vi "usrp_tx.vi"() -> ()   [LabVIEW 2014]
uses:
  <vilib>/addons/Modulation/Analog/support/mod_Set Error Source.vi
  var_stop.vi
  <vilib>/addons/Modulation/Digital/Support/Common/Validators/mod_Generate Filter Coefficients Validate.vi
  <vilib>/addons/Modulation/Digital/General/subVIs/mod_Generate Filter Coefficients.vi
  <vilib>/addons/Modulation/Digital/General/MT Apply Pulse Shaping Filter (Generic).vi
  <instrlib>/niUSRP/niUSRP Write Tx Data (CDB Cluster).vi
  <vilib>/addons/Modulation/niDMT.lvlib
panel:
  out "error out":errorcluster
  in  "DPSK type":enum16{"binary", "quadrature"}(ring)=enum."quadrature"
  in  "Send Text":bool
  in  "Text to send":string="This is a point-to-point link prototype with synchronization algorithm implemented and is developed by Teng-Hui Huang, Netwrok  Information and Communications Laboratory, NTU Taiwan.\n\nQuick start:\n1. Connect your PC to a USRP.\n2. Run usrp_tx.vi.\n3. Run usrp_rx.vi.\n4. Press \"Send Text\"\n\nFor any issues please send me an e-mail:\nhui811116@outlook.com\n\nTeng-Hui Huang\n2017.11.19"
  in  "System Stop":bool
  in  "Enabled Channels":string(combo)="0"
  in  "Timebase Clock Source":string(combo)="Internal"
  in  "Frequency Source":string(combo)="Internal"
  out "coerced gain":dbl format="%#_6f"
  out "coerced carrier frequency":dbl=100000.0 format="%#_6p"
  out "coerced IQ rate":dbl=100000.0 format="%#_6p"
  in  "active antenna":string="TX1"
  in  "gain":dbl=10.0 format="%#_6f"
  in  "carrier frequency":dbl=915000000.0 format="%#_6p"
  in  "device names":refnum<k15>="192.168.10.3"
  in  "IQ rate":dbl=1000000.0 format="%#_6p"
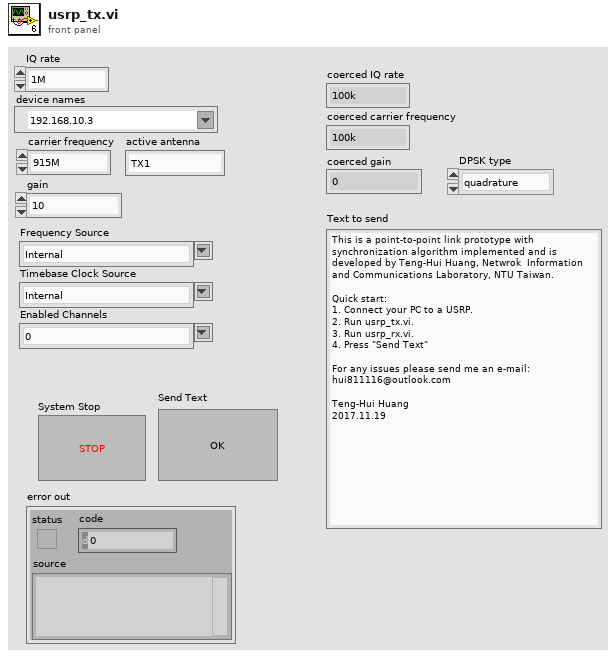
[diagram p1: front panel]
types:
  T1 = enum16{"none", "Raised Cosine", "Root Raised Cos", "Gaussian"}
  T2 = enum16{"FSK", "PSK", "QAM", "MSK", "PAM", "ASK", "CPM"}
  T3 = typedef "niAMT.lvlib/Complex Data Waveform.ctl" = cluster{"t0":dbl, "dt":dbl, "Y":cdb[]}
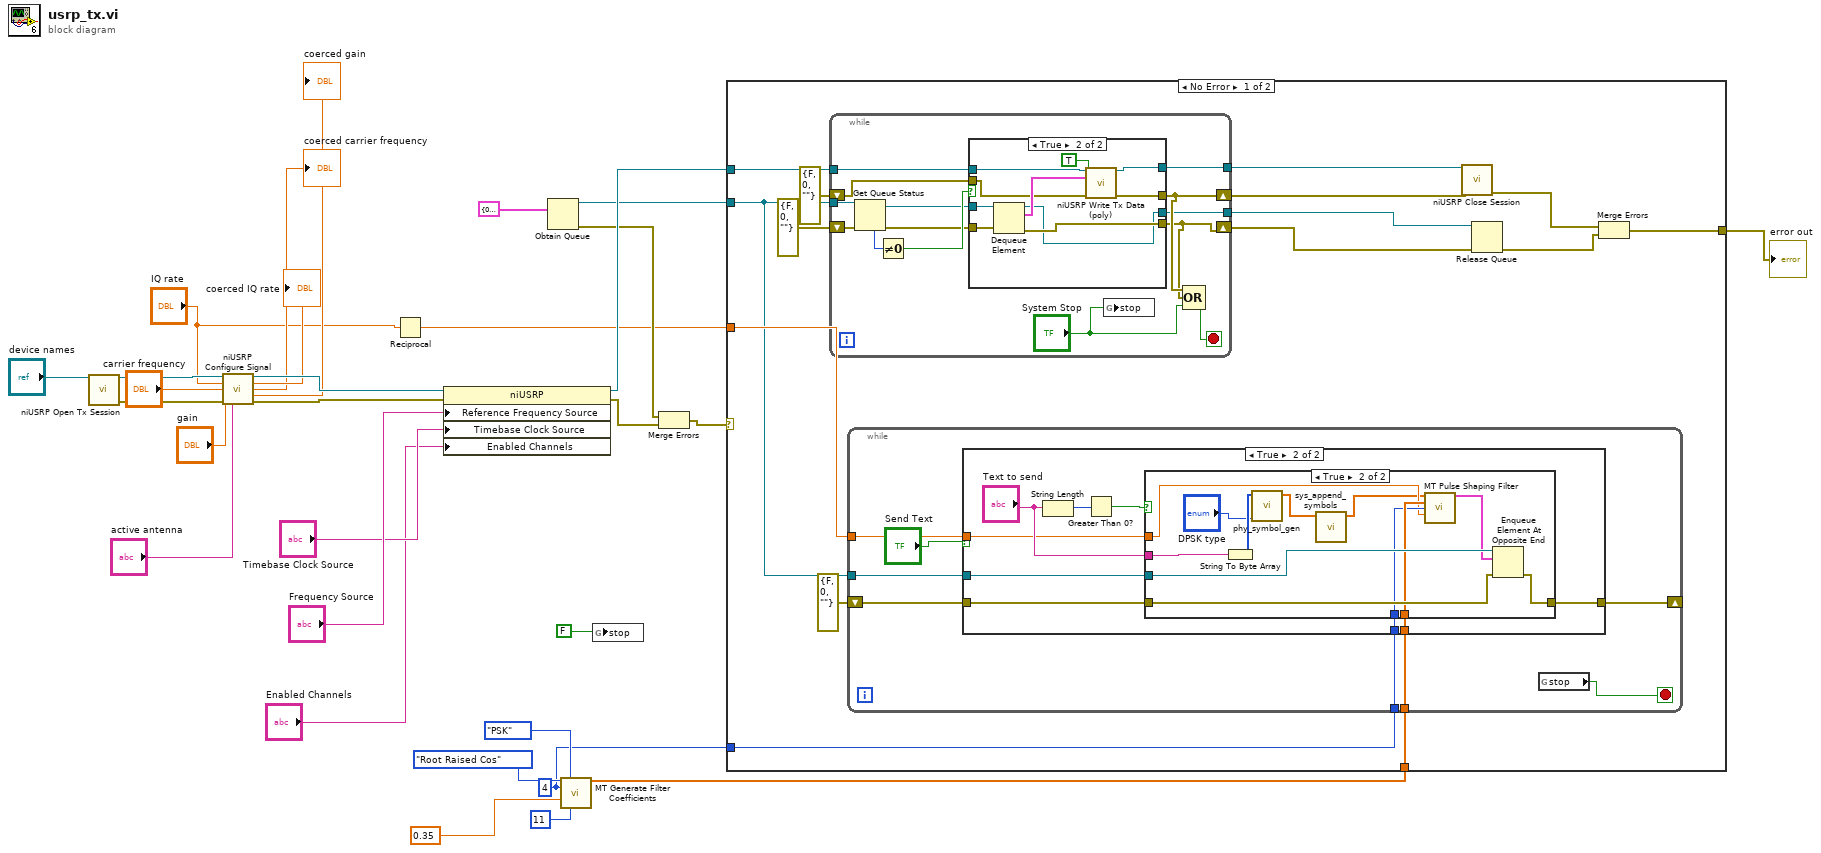
[diagram p0: block diagram]
diagram:
  w2 = 4 ("pulse shaping samples per symbol (16)")
  n1 = call <instrlib>:"niUSRP Open Tx Session.vi"("device names"="device names") -> ("session handle out"=w30:refnum<k15>, "error out"=w29:errorcluster)  [unwired: 13 in]
  n2 = call <instrlib>:"niUSRP Configure Signal.vi"("session handle"=w30, "IQ rate"="IQ rate", "carrier frequency"="carrier frequency", "gain"="gain", "error in (no error)"=w29, "active antenna"="active antenna") -> ("session handle out"=w24:refnum<k15>, "coerced IQ rate"=→"coerced IQ rate":dbl, "coerced carrier frequency"=→"coerced carrier frequency":dbl, "coerced gain"=→"coerced gain":dbl, "error out"=w23:errorcluster)  [unwired: 5 in]
  n3 = Reciprocal(x="IQ rate") -> (1/x=w9:dbl)
  n4 = property class="niUSRP"(reference=w24, error in=w23, "Reference Frequency Source"="Frequency Source", "Timebase Clock Source"="Timebase Clock Source", "Enabled Channels"="Enabled Channels") -> (reference out=w16:refnum<k15>, error out=w14:errorcluster)
  n5 = Obtain Queue(element data type=cluster{"t0":dbl, "dt":dbl, "Y":cdb[]} {"t0"=0.0, "dt"=1.0, "Y"=[]} ("data")) -> (queue out=w15:refnum<queue>, error out=w13:errorcluster)  [unwired: 4 in, 1 out]
  n6 = call <vilib>:"MT Generate Filter Coefficients.vi"("pulse shaping filter (none)"=T1."Root Raised Cos", "modulation type"=T2."PSK", "pulse shaping samples per symbol (16)"=w2, "filter parameter"=0.35, "filter length (symbols)"=11) -> ("pulse shaping filter coefficients"=w3:dbl[])  [unwired: 8 in, 2 out]
  n7 = global write "var_stop.vi" "stop"(FALSE) -> ()
  n8 = Merge Errors(w13, w14) -> (w12:errorcluster)
  n9 = case shown="No Error" w12 {
    selector: w12 -> [_ w105]
    tunnel: w16 -> [w45 _]
    tunnel: w15 -> [w36 _]
    tunnel: w9 -> [w38 _]
    tunnel: w3 -> [w35 _]
    tunnel: w2 -> [w34 _]
    tunnel: [w31 w105] -> w1
    frame No Error {
      n10 = while {
        tunnel: w45 -> [w84]
        tunnel: w36 -> [w89]
        shift-right: [w80] -> w40
        shift-left: errorcluster {"status"=FALSE, "code"=0, "source"=""} ("error out") -> [w88]
        tunnel: [w83] -> w44
        shift-right: [w81] -> w43
        shift-left: errorcluster {"status"=FALSE, "code"=0, "source"=""} ("error out") -> [w82]
        tunnel: [w78] -> w39
        stop <- w79 stop-if-true
        n11 = Get Queue Status(queue=w89, error in (no error)=w88) -> (queue out=w86:refnum<queue>, error out=w85:errorcluster, # elements in queue=w90:i32)  [unwired: 1 in, 5 out]
        n12 = Not Equal To 0?(x=w90) -> (x != 0?=w87:bool)
        n13 = case shown="True" w87 {
          tunnel: w86 -> [w91 w104]
          tunnel: w85 -> [w94 w103]
          tunnel: [w94 w102] -> w80
          tunnel: w84 -> [w93 w100]
          tunnel: [w93 w99] -> w83
          tunnel: [w92 w98] -> w81
          tunnel: w82 -> [w92 w97]
          tunnel: [w91 w95] -> w78
          frame False {
          }
          frame True {
            n14 = Dequeue Element(queue=w104, error in (no error)=w103) -> (queue out=w95:refnum<queue>, element=w101:cluster{"t0":dbl, "dt":dbl, "Y":cdb[]}, error out=w102:errorcluster)  [unwired: 1 in, 1 out]
            n15 = call-poly <instrlib>:"niUSRP Write Tx Data (poly).vi"("session handle"=w100, "data"=w101, "end of data?"=TRUE, "error in (no error)"=w97) -> ("session handle out"=w99:refnum<k15>, "error out"=w98:errorcluster)  [unwired: 10 in]
          }
        }
        n16 = global write "var_stop.vi" "stop"("System Stop") -> ()
        n17 = Compound Arithmetic op=OR(w81, w80, "System Stop") -> (w79:bool)
      }
      n18 = while {
        tunnel: w38 -> [w52]
        shift-right: [w50] -> _
        shift-left: errorcluster {"status"=FALSE, "code"=0, "source"=""} ("error out") -> [w51]
        tunnel: w36 -> [w49]
        tunnel: w35 -> [w47]
        tunnel: w34 -> [w46]
        stop <- w48 stop-if-true
        n19 = case shown="True" "Send Text" {
          tunnel: w52 -> [_ w60]
          tunnel: w51 -> [w54 w59]
          tunnel: [w54 w58] -> w50
          tunnel: w49 -> [_ w57]
          tunnel: w47 -> [_ w56]
          tunnel: w46 -> [_ w55]
          frame False {
          }
          frame True {
            n20 = String Length(string="Text to send") -> (length=w63:i32)
            n21 = Greater Than 0?(x=w63) -> (x > 0?=w62:bool)
            n22 = case shown="True" w62 {
              tunnel: "Text to send" -> [_ w76]
              tunnel: w57 -> [_ w75]
              tunnel: w60 -> [_ w68]
              tunnel: w59 -> [w64 w73]
              tunnel: [w64 w72] -> w58
              tunnel: w56 -> [_ w70]
              tunnel: w55 -> [_ w69]
              frame False {
              }
              frame True {
                n23 = String To Byte Array(string=w76) -> (unsigned byte array=w74:u8[])
                n24 = call "phy_symbol_gen.vi"("type"="DPSK type", "Input bytes"=w74) -> ("symbols"=w66:cdb[])  [unwired: 9 in]
                n25 = call "sys_append_symbols.vi"("raw symbols"=w66) -> ("appended symbols"=w65:cdb[])  [unwired: 10 in]
                n26 = call-poly <vilib>:"MT Pulse Shaping Filter.vi"("symbols"=w65, "pulse shaping filter coefficients"=w70, "samples per symbol (16)"=w69, "symbol rate (Hz)"=w68) -> ("output complex waveform"=w67:T3)  [unwired: 10 in, 1 out]
                n27 = Enqueue Element At Opposite End(queue=w75, element=w67, error in (no error)=w73) -> (error out=w72:errorcluster)  [unwired: 1 in, 2 out]
              }
            }
          }
        }
        n28 = global read "var_stop.vi" "stop"() -> (w48:bool)
      }
      n29 = call <instrlib>:"niUSRP Close Session.vi"("session handle"=w44, "error in (no error)"=w43) -> ("error out"=w33:errorcluster)  [unwired: 13 in]
      n30 = Release Queue(queue=w39, error in (no error)=w40) -> (error out=w32:errorcluster)  [unwired: 1 in, 2 out]
      n31 = Merge Errors(w33, w32) -> (w31:errorcluster)
    }
    frame Error {
    }
  }
  "error out" <- w1
